vi "IFA300ErrorCodes.vi"(4 "Error Code":string) -> (1 "Error Description":string)   [LabVIEW 2011]
panel:
  out "Array 2":string[](array[string])
  out "Array":string[](array[string])
  in  "IFA300 Error Strings":string="-100 INST Base command syntax error. \n-101 Channel number is not valid. \n-102 Attempt to access board not installed. \n-110 CONF Base command syntax error. \n-111 Set gain on channel failed. \n-112 Set offset voltage failed. \n-113 Set probe type failed. \n-114 Set of resistor value failed. \n-115 Set cable length failed. \n-116 Set hi power bridge failed. \n-117 Setting overheat ratio failed. \n-120 READ Base command syntax error. \n-121 Read of 8-bit a/d produced an invalid number. \n-122 Xmit of last temp value failed. \n-130 MEAS Base command syntax error. \n-131 Measure resistance failed. \n-132 Measure temp with 12-bit failed. \n-140 INIT Base command syntax error. \n-141 Missing channel number on command line. \n-142 Channel already is already in run mode. \n-143 Stop a channel that is not running. \n-144 High-power bridge is selected with a wire probe type. This is not allowed. \n-150 TEST Base command syntax error. \n-151 Processing test command failed. \n-160 STAT Base command syntax error. \n-170 OUTP Base command syntax error. \n-171 Set high pass filter failed. \n-172 Set low pass filter failed. \n-173 Invalid channel. \n-300 Invalid command received. Second level command syntax error. \n-301 No anemometer boards detected at power on. \n-303 A channel is indicating a FAULT condition. \n-304 An invalid channel was read at power on. \n"
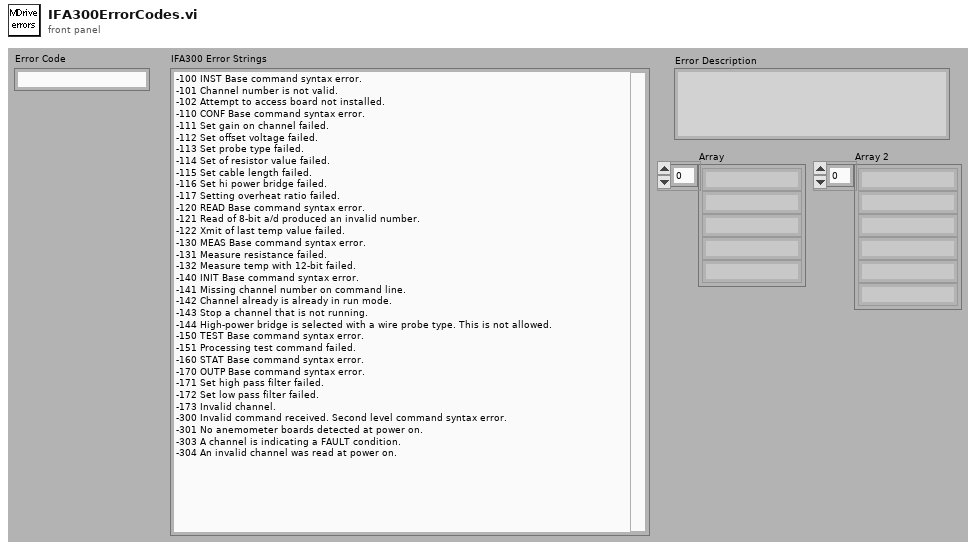
[diagram p1: front panel]
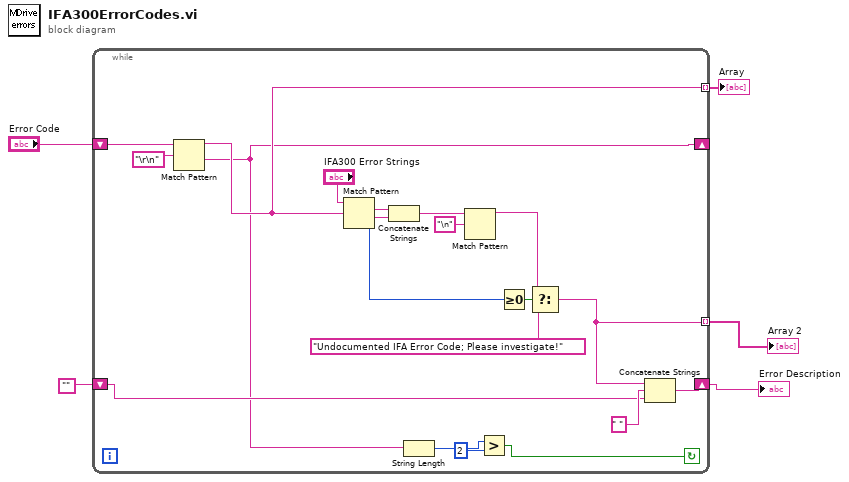
[diagram p0: block diagram]
diagram:
  n1 = while {
    shift-right: [w9] -> _
    shift-left: "Error Code" -> [w15]
    shift-right: [w16] -> w1
    shift-left: "" -> [w11]
    tunnel: [w13] -> w3 mode=indexing
    tunnel: [w10] -> w2 mode=indexing
    stop <- w7 continue-if-true
    n2 = Match Pattern(string=w15, regular expression="\r\n") -> (before substring=w13:string, after substring=w9:string)  [unwired: 3 out]
    n3 = Match Pattern(string="IFA300 Error Strings", regular expression=w13) -> (match substring=w23:string, after substring=w22:string, offset past match=w20:i32)  [unwired: 2 out]
    n4 = Concatenate Strings(w23, w22) -> (w21:string)
    n5 = String Length(string=w9) -> (length=w8:i32)
    n6 = Match Pattern(string=w21, regular expression="\n") -> (before substring=w18:string)  [unwired: 4 out]
    n7 = Greater?(x=w8, y=2) -> (0:w7:bool)
    n8 = Greater Or Equal To 0?(x=w20) -> (x >= 0?=w19:bool)
    n9 = Select(t=w18, s=w19, f="Undocumented IFA Error Code; Please investigate!") -> (s? t:f=w10:string)
    n10 = Concatenate Strings(w10, " " ("string"), w11) -> (w16:string)
  }
  "Array" <- w3
  "Array 2" <- w2
  "Error Description" <- w1
